vi "Elapsed time in seconds between two dates.vi"(0 "Start Date/Time":string="12-Mar-2018 11:55:33", 2 "End Date/Time":string="12-Mar-2018 11:55:33") -> (7 "Time difference in Seconds":string)   [LabVIEW 2019]
doc: "Elapsed time in seconds between 2 dates"
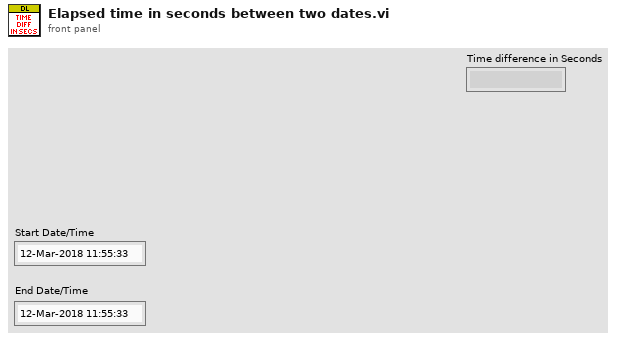
[diagram p1: front panel]
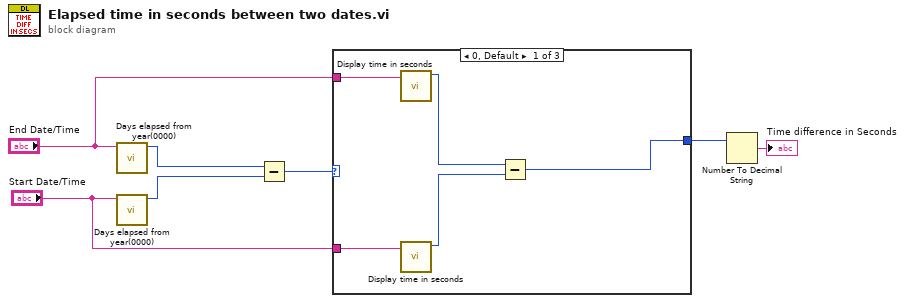
[diagram p0: block diagram]
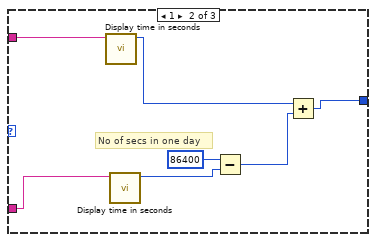
[diagram p2: hidden frame]
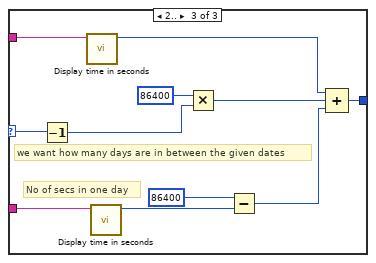
[diagram p3: hidden frame]
diagram:
  n1 = call "Days elapsed from year(0000).vi"("Date/Time"="End Date/Time") -> ("No of days passed from the date(00/00/0000)"=w7:i32)  [unwired: 10 in]
  n2 = call "Days elapsed from year(0000).vi"("Date/Time"="Start Date/Time") -> ("No of days passed from the date(00/00/0000)"=w6:i32)  [unwired: 10 in]
  n3 = Subtract(x=w7, y=w6) -> (x-y=w5:i32)
  n4 = case shown="0, Default" w5 {
    selector: w5 -> [_ _ w23]
    tunnel: "End Date/Time" -> [w12 w15 w28]
    tunnel: "Start Date/Time" -> [w11 w19 w27]
    tunnel: [w8 w13 w20] -> w2
    frame 0, Default {
      n5 = call "Display time in seconds.vi"("Event Date/Time"=w12) -> ("Time in Seconds"=w10:i32)  [unwired: 10 in]
      n6 = call "Display time in seconds.vi"("Event Date/Time"=w11) -> ("Time in Seconds"=w9:i32)  [unwired: 10 in]
      n7 = Subtract(x=w10, y=w9) -> (x-y=w8:i32)
    }
    frame 1 {
      # "No of secs in one day"
      n8 = call "Display time in seconds.vi"("Event Date/Time"=w15) -> ("Time in Seconds"=w14:i32)  [unwired: 10 in]
      n9 = call "Display time in seconds.vi"("Event Date/Time"=w19) -> ("Time in Seconds"=w18:i32)  [unwired: 10 in]
      n10 = Subtract(x=86400, y=w18) -> (x-y=w16:i32)
      n11 = Add(x=w14, y=w16) -> (x+y=w13:i32)
    }
    frame 2.. {
      # "we want how many days are in between the given dates"
      # "No of secs in one day"
      n12 = Decrement(x=w23) -> (x-1=w22:i32)
      n13 = call "Display time in seconds.vi"("Event Date/Time"=w28) -> ("Time in Seconds"=w26:i32)  [unwired: 10 in]
      n14 = call "Display time in seconds.vi"("Event Date/Time"=w27) -> ("Time in Seconds"=w30:i32)  [unwired: 10 in]
      n15 = Multiply(x=86400, y=w22) -> (x*y=w21:i32)
      n16 = Subtract(x=86400, y=w30) -> (x-y=w25:i32)
      n17 = Compound Arithmetic op=ADD(w26, w21, w25) -> (w20:i32)
    }
  }
  n18 = Number To Decimal String(number=w2) -> (decimal integer string=→"Time difference in Seconds":string)  [unwired: 1 in]
